vi "Disable Default File.vi"(8 "Error In":errorcluster) -> (0 "Error Out":errorcluster)   [LabVIEW 2014, in "LV-Logger.lvlib"]
uses:
  LV-Logger.lvlib
  Private/_File Manager Action.ctl
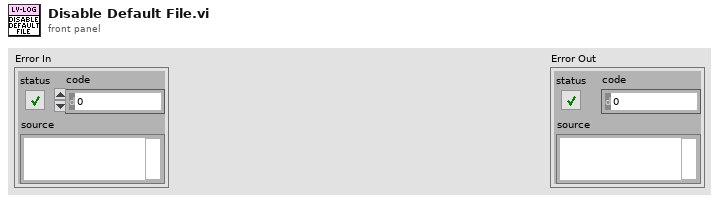
[diagram p1: front panel]
types:
  T1 = typedef "LV-Logger.lvlib/_File Manager Action.ctl" = enum16{"Initialize", "Set File Size Limit", "Set Root Folder", "Set Application Name", "Start", "Write", "Stop", "Shutdown"}
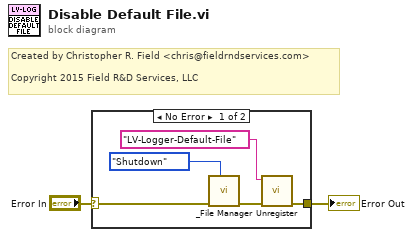
[diagram p0: block diagram]
diagram:
  # "Created by Christopher R. Field <chris@fieldrndservices.com>\n\nCopyright 2015 Field R&D Services, LLC"
  n1 = case shown="No Error" "Error In" {
    selector: "Error In" -> [w6 w8]
    tunnel: [w5 w8] -> w1
    frame No Error {
      n2 = call "_File Manager.vi"("Action"=_File_Manager_Action."Shutdown", "Error In"=w6) -> ("Error Out"=w4:errorcluster)  [unwired: 9 in]
      n3 = call "Unregister.vi"("Error In"=w4, "Listener ID"="LV-Logger-Default-File") -> ("Error Out"=w5:errorcluster)  [unwired: 9 in]
    }
    frame Error {
    }
  }
  "Error Out" <- w1
